vi "Form Coordinates.vi"(0 "Palette Item Icon":T2[](array[typedef]), 9 "No.of Elements in Row":i32=3) -> (4 "Co-ordinates":T1(array[cluster]))   [LabVIEW 2014, in "SmartPalette.lvlib"]
uses:
  SmartPalette.lvlib
  <vilib>/picture/picture.llb/imagedata.ctl
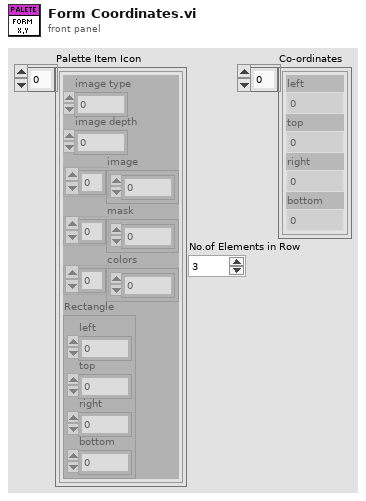
[diagram p1: front panel]
types:
  T1 = cluster{"left":i16, "top":i16, "right":i16, "bottom":i16}[]
  T2 = typedef "imagedata.ctl" = cluster{"image type":i32, "image depth":i32, "image":u8[], "mask":u8[], "colors":u32[], "Rectangle":cluster{"left":i16, "top":i16, "right":i16, "bottom":i16}}
  T3 = cluster{"left":i16, "top":i16, "right":i16, "bottom":i16}
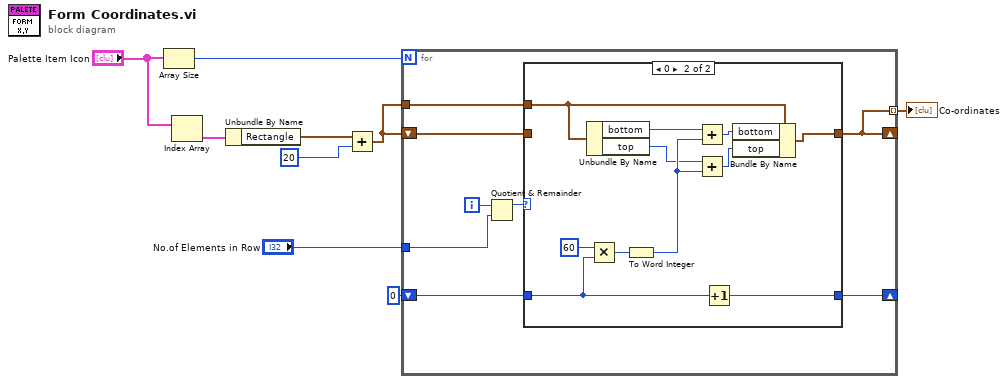
[diagram p0: block diagram]
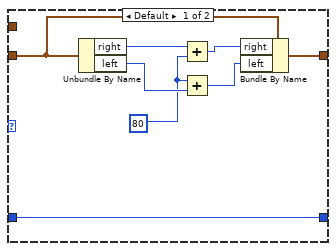
[diagram p2: hidden frame]
diagram:
  n1 = Array Size(array="Palette Item Icon") -> (size(s)=w8:i32)
  n2 = Index Array(array="Palette Item Icon") -> (element=w9:T2)  [unwired: 1 in]
  n3 = Unbundle By Name(w9) -> ("Rectangle"=w6:T3)
  n4 = Add(x=w6, y=i16 20) -> (x+y=w4:T3)
  n5 = for {
    N: w8 -> [_]
    shift-right: [w14] -> _
    shift-left: w4 -> [w15]
    tunnel: [w14] -> w2 mode=indexing
    tunnel: w4 -> [w11]
    shift-right: [w12] -> _
    shift-left: 0 -> [w13]
    tunnel: "No.of Elements in Row" -> [w10]
    i -> [w17]
    n6 = Quotient & Remainder(x=w17, y=w10) -> (x-y*floor(x/y)=w16:i32)  [unwired: 1 out]
    n7 = case shown="0" w16 {
      tunnel: w15 -> [w25 _]
      tunnel: [w21 w33] -> w14
      tunnel: w13 -> [w20 w32]
      tunnel: [w20 w31] -> w12
      tunnel: w11 -> [_ w35]
      frame Default {
        w18 = i16 80
        n8 = Unbundle By Name(w25) -> ("right"=w19:i16, "left"=w23:i16)
        n9 = Add(x=w19, y=w18) -> (x+y=w24:i16)
        n10 = Add(x=w18, y=w23) -> (x+y=w22:i16)
        n11 = Bundle By Name(cluster=w25, "right"=w24, "left"=w22) -> (w21:T3)
      }
      frame 0 {
        n12 = Unbundle By Name(w35) -> ("bottom"=w26:i16, "top"=w28:i16)
        n13 = Multiply(x=60, y=w32) -> (x*y=w34:i32)
        n14 = To Word Integer(number=w34) -> (16bit integer=w29:i16)
        n15 = Add(x=w26, y=w29) -> (x+y=w30:i16)
        n16 = Add(x=w28, y=w29) -> (x+y=w27:i16)
        n17 = Increment(x=w32) -> (x+1=w31:i32)
        n18 = Bundle By Name(cluster=w35, "bottom"=w30, "top"=w27) -> (w33:T3)
      }
    }
  }
  "Co-ordinates" <- w2
